vi "Get_ADODB._Connection.vi"(8 "error in (no error)":errorcluster caption="错误输入（无错误）", 11 "Database Recordset输入":refnum<class "Database Recordset.lvclass">) -> (0 "error out":errorcluster caption="错误输出", 2 "ADODB._Connection":refnum<k7>, 3 "Database Recordset输出":refnum<class "Database Recordset.lvclass">)   [LabVIEW 2011, in "Database Recordset.lvclass"]
uses:
  Database Recordset.lvclass
  Database Recordset.lvclass/Database Recordset.ctl
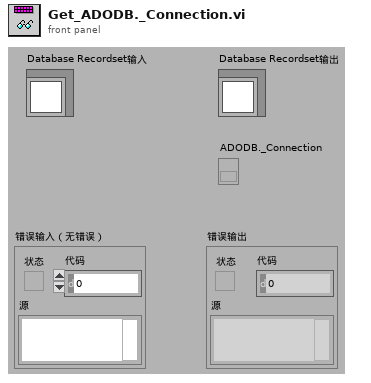
[diagram p1: front panel]
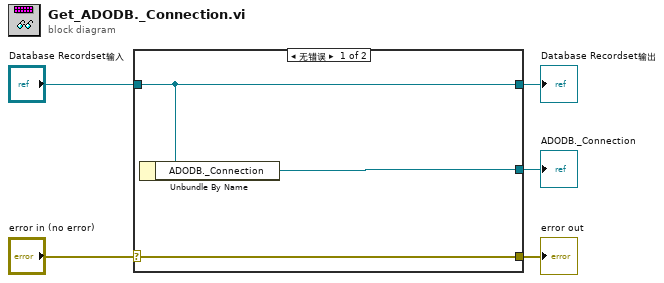
[diagram p0: block diagram]
diagram:
  n1 = case shown="无错误" "error in (no error)" {
    selector: "error in (no error)" -> [w8 w9]
    tunnel: [w8 w9] -> w4
    tunnel: [w7 w10] -> w2
    tunnel: "Database Recordset输入" -> [w7 w10]
    tunnel: [w6 _] -> w1
    frame No Error {
      n2 = Unbundle By Name(w7) -> ("ADODB._Connection"=w6:refnum<k7>)
    }
    frame Error {
    }
  }
  "error out" <- w4
  "Database Recordset输出" <- w2
  "ADODB._Connection" <- w1
